vi "UHR-Fleezers Control (host) - Lorentz v5.vi"() -> ()   [LabVIEW 2014] (continued)
    n2967 = xnode "Get APD Data"("FPGA VI Reference In"=w4409, "error in"=w4408, "Number of Elements"=w4314, "Timeout (ms)"=-1) -> ("Data"=w4229:u32[], "Elements Remaining"=→"APD FIFO Elements Remaining":u32)  [unwired: 2 out]
    n2968 = feedback #1(0.0) -> (w4400:dbl)
    n2969 = To Time Stamp(1:w4400) -> (0:w4212:timestamp)
    n2970 = Add(x=w4235, y=w4400) -> (x+y=w4488:dbl)
    n2971 = feedback-in #1(w4488) -> ()
    n2972 = Subtract(x=w4513, y=w4444) -> (x-y=w4512:u32)
    n2973 = local read "APD Integration Time (s)"() -> (w4221:dbl)
    n2974 = Divide(x=w4511, y=w4512) -> (x/y=w4510:dbl)
    "Buffer Status" <- w4510
    n2975 = local read "Trap Sets"() -> (w4240:u32)
    n2976 = Equal?(x=w4510, y=1.0) -> (x = y?=w4508:bool)
    n2977 = local read "Number of APDs"() -> (w4228:u8)
    n2978 = Decimate 1D Array(w4377) -> (w4374:u16[], w4376:u16[], w4375:u16[], w4219:u16[], w4217:u16[])
    n2979 = case "Alert buffer overflow" shown="True" w4508 {
      frame False {
      }
      frame True {
        n2980 = call <vilib>:"Beep.vi"() -> ()  [unwired: 3 in, 9 out]
        "Overflow (data lost)" <- TRUE ("Overflow (data lost)")
      }
    }
    n2981 = To Unsigned Long Integer(number=w4374) -> (unsigned 32bit integer=w4373:u32[])
    n2982 = Join Numbers(hi=w4376, lo=w4375) -> ((hi.lo)=w4372:u32[])
    n2983 = Divide(x=w4219, y=w4218) -> (x/y=w4200:dbl[])
    n2984 = Divide(x=w4217, y=w4218) -> (x/y=w4199:dbl[])
    n2985 = call "deinterlace.vi"("Detector type"="Detector Type", "Data"=w4239, "Trap sets"=w4240, "Flip x sign"="Flip X Sign") -> ("Channel pattern"=w4236:i32, "Channel names"=w4172:string[], "Deinterlaced normalized data"=w4233:dbl[][], "Deinterlaced data"=w4237:i16[])
    "AI labels" <- w4172
    n2986 = Join Numbers(hi=w4373, lo=w4372) -> ((hi.lo)=w4367:u64[])
    n2987 = local read "Data Period (s)"() -> (w4206:dbl)
    n2988 = call "APD data extraction.vi"("Data"=w4229, "Number of APD's"=w4228, "APD integration time (s)"=w4221, "APD Ave N"="APD Ave N", "APD Disp. Downsample"="APD Disp. Downsample", "APD Disp. Scale"="APD Disp. Scale", "Time Stamp"=w4212) -> ("Output cluster"=→"APD rates cluster":T1, "Output Data"=w4224:T59, "Output waveform"=w4223:waveform(dbl)[], "APD Display period (s)"=w4222:dbl)
    "APD Display Period (s)" <- w4222
    n2989 = call "IR AOM word to freq - vec.vi"("Frequency Word In (double vec)"=w4367) -> ("Frequency Out"=w4404:dbl[])
    n2990 = Decimate 1D Array(w4199) -> (w4196:dbl[], w4195:dbl[])
    n2991 = Decimate 1D Array(w4200) -> (w4198:dbl[], w4197:dbl[])
    n2992 = Add(x=w4198, y=w4197) -> (x+y=w4194:dbl[])
    n2993 = Add(x=w4196, y=w4195) -> (x+y=w4193:dbl[])
    n2994 = Decimate 1D Array(w4404) -> (w4403:dbl[], w4402:dbl[])
    n2995 = Divide(x=w4194, y=w4192) -> (x/y=w4190:dbl[])
    n2996 = Divide(x=w4193, y=w4192) -> (x/y=w4191:dbl[])
    n2997 = Reciprocal(x=w4222) -> (1/x=→"APD Display Freq. (Hz)":dbl)
    n2998 = Build Array(w4403, w4402, w4190, w4191) -> (w4213:dbl[][])
    n2999 = Multiply(x=w4206, y="Trap Disp. Downsample") -> (x*y=w4401:dbl)
    "Display Period (s)" <- w4401
    n3000 = for {
      tunnel: w4233 -> [w4556] mode=indexing
      tunnel: [w4555] -> w4171 mode=indexing
      n3001 = call-poly <vilib>:"Mean.vi"("X"=w4556) -> ("mean"=w4555:dbl)  [unwired: 1 out]
    }
    "Values" <- w4171
    n3002 = call "Generate Waveform.vi"("Downsampling"="Trap Disp. Downsample", "Data Period (s)"=w4206, "Data"=w4233, "Plot names"=w4172, "Time Stamp"=w4212) -> ("Downsampled data"=w4231:waveform(dbl)[], "Non downsampled waveform"=w4230:waveform(dbl)[])
    n3003 = Multiply(x="APD Disp. Scale", y=w4223) -> (x*y=w4422:waveform(dbl)[])
    n3004 = Reciprocal(x=w4401) -> (1/x=→"Trap Disp. Freq. (Hz)":dbl)
    n3005 = Multiply(x="APD Disp. Downsample", y=w4221) -> (x*y=w4421:dbl)
    n3006 = Decimate 1D Array(w4237) -> (w4392:i16[], w4391:i16[], w4389:i16[], w4388:i16[])  [unwired: 9 out]
    n3007 = Divide(x=w4422, y=w4421) -> (x/y=w4319:waveform(dbl)[])
    n3008 = case shown="1" "Plot Trap Positions" {
      tunnel: [w4541 w4550] -> w4207
      frame 0, Default {
        n3009 = local read "BD 1 Frequency 2 (MHz)"() -> (w4544:dbl)
        n3010 = local read "BD 1 Frequency 1 (MHz)"() -> (w4545:dbl)
        n3011 = local read "T3 Y (V)"() -> (w4542:dbl)
        n3012 = local read "T3 X (V)"() -> (w4543:dbl)
        n3013 = Build Array(w4545, w4544, w4543, w4542) -> (w4541:dbl[])
      }
      frame 1 {
        w4549 = 75.0
        n3014 = Unbundle By Name("Piezo trap 0 position relative to 75 MHz") -> ("X (V)"=w4547:dbl, "Y (V)"=w4546:dbl)
        n3015 = Build Array(w4549, w4549, w4547, w4546) -> (w4550:dbl[])
      }
    }
    n3016 = Divide(x=w4392, y=w4391) -> (x/y=w4393:dbl[])
    n3017 = Divide(x=w4389, y=w4388) -> (x/y=w4390:dbl[])
    n3018 = local read "AOM X Cal (nm/MHz)"() -> (w4209:dbl)
    n3019 = Split 1D Array(array=w4393, index="N El. to Ave.") -> (second subarray=w4396:dbl[])  [unwired: 1 out]
    n3020 = Split 1D Array(array=w4390, index="N El. to Ave.") -> (second subarray=w4395:dbl[])  [unwired: 1 out]
    n3021 = Index Array(array=w4319, index=0) -> (element=w4417:waveform(dbl))
    n3022 = Index Array(array=w4319, index=1) -> (element=w4415:waveform(dbl))
    n3023 = Index Array(array=w4319, index=2) -> (element=w4321:waveform(dbl))
    n3024 = call-poly <vilib>:"Mean.vi"("X"=w4396) -> ("mean"=w4384:dbl)  [unwired: 1 out]
    n3025 = call-poly <vilib>:"Mean.vi"("X"=w4395) -> ("mean"=w4383:dbl)  [unwired: 1 out]
    n3026 = Subtract(x=w4417, y="APD 1 Offset") -> (x-y=w4413:waveform(dbl))
    n3027 = Subtract(x=w4415, y="APD 2 Offset") -> (x-y=w4412:waveform(dbl))
    n3028 = Subtract(x=w4321, y="APD 3 Offset") -> (x-y=w4318:waveform(dbl))
    n3029 = Build Array(w4413, w4412, w4318) -> (→"APD Chart":waveform(dbl)[])
    n3030 = Build Array(w4209, w4209, "Piezo Trap X cal (nm/V)", "Piezo Trap Y cal (nm/V)") -> (w4208:dbl[])
    n3031 = local read "Trap X AI1 (DMA)"() -> (w4394:T19)
    n3032 = To Fixed-Point(number=w4383) -> (fixed-point=w4381:fxp<+/-,16,1>)  [unwired: 1 in]
    n3033 = To Fixed-Point(number=w4384) -> (fixed-point=w4382:fxp<+/-,16,1>)  [unwired: 1 in]
    n3034 = Cluster To Array(cluster="Negate Axis") -> (array=w4201:bool[])
    n3035 = call "Generate Trap Positiion Waveform.vi"("Base trap positions"=w4207, "Data Period (s)"=w4206, "Input data"=w4213, "Position calibration values"=w4208, "Trap Pos. Disp. Downsample (s)"="Trap Pos. Disp. Downsample", "Negate axis"=w4201, "Time Stamp"=w4212) -> ("Output waveforms"=w4178:waveform(dbl)[])  [unwired: 3 in]
    "Trap Positions" <- w4178
    n3036 = Bundle By Name(cluster=w4394, "Set 1"=w4382, "Set 2"=w4381) -> (→"Trap X AI1 (DMA)":T19)
    n3037 = Initialize Array(0.0) -> (w4203:dbl[][])  [unwired: 2 in]
    n3038 = local read "Display Period (s)"() -> (w4431:dbl)
    n3039 = for {
      tunnel: w4178 -> [w4554] mode=indexing
      shift-right: [w4552] -> w4180
      shift-left: w4203 -> [w4553]
      n3040 = Unbundle By Name(w4554) -> ("Y"=w4551:dbl[])
      n3041 = Build Array (concatenate)(w4553, w4551) -> (w4552:dbl[][])
    }
    n3042 = Build Array (concatenate)(w4223, w4231) -> (w4234:waveform(dbl)[])
    "All Signals" <- w4234
    n3043 = Divide(x="Bead Sep. Int. Time (s)", y=w4431) -> (x/y=w4186:dbl)
    n3044 = feedback #2(w4180) -> (w4187:dbl[][])
    n3045 = call "Trap Pos RMS.vi"("Accumulated array"=w4187, "New Array"=w4180, "Number of sets to average"=w4186) -> ("Output accumulated array"=w4185:dbl[][], "RMS"=w4183:dbl[], "Mean"=w4184:dbl[])
    n3046 = feedback-in #2(w4185) -> ()
    n3047 = Index Array(array=w4180, index (row)=0 ("index")) -> (element=w4179:dbl[])  [unwired: 1 in]
    n3048 = Array To Cluster(array=w4183) -> (cluster=→"Trap RMS (ang)":T60)
    n3049 = Array To Cluster(array=w4184) -> (cluster=→"Mean Trap Positions (nm)":T61)
    n3050 = local read "Data points/scans (MCL)"() -> (w4471:dbl)
    n3051 = Unbundle(w4224) -> ("APD 1"=w4317:u32[])  [unwired: 2 out]
    n3052 = To Double Precision Float(number=w4317) -> (double precision float=w4439:dbl[])
    n3053 = Increment(x=w4471) -> (x+1=w4472:dbl)
    n3054 = feedback #3(w4472) -> (w4475:dbl)
    n3055 = Select(t=0, s=w4462, f=w4475) -> (s? t:f=w4468:dbl)
    n3056 = Array Size(array=w4439) -> (size(s)=w4474:i32)
    n3057 = Add(x=w4474, y=w4468) -> (x+y=w4469:dbl)
    n3058 = Greater?(x=w4469, y=w4471) -> (0:w4470:bool)
    n3059 = Select(t=w4468, s=w4470, f=w4469) -> (s? t:f=w4467:dbl)
    n3060 = feedback-in #3(w4467) -> ()
    n3061 = local read "MCL Scanning"() -> (w4465:bool)
    n3062 = Index Array(array=w4231, index="index 1") -> (element=w4309:waveform(dbl))
    n3063 = Index Array(array=w4231, index="index 2") -> (element=w4313:waveform(dbl))
    n3064 = Unbundle By Name(w4309) -> ("Y"=w4308:dbl[])
    n3065 = Unbundle By Name(w4313) -> ("Y"=w4312:dbl[])
    n3066 = Not(x=w4470) -> (.not. x?=w4464:bool)
    n3067 = And(x=w4464, y=w4465) -> (x .and. y?=w4466:bool)
    n3068 = call-poly <vilib>:"Mean.vi"("X"=w4308) -> ("mean"=→"Trap 1 sum mean":dbl)  [unwired: 1 out]
    n3069 = call-poly <vilib>:"Mean.vi"("X"=w4312) -> ("mean"=→"Trap 2 sum mean":dbl)  [unwired: 1 out]
    n3070 = Or(x=w4466, y=w4462) -> (x .or. y?=w4463:bool)
    n3071 = Equal?(x="Tab Control 6", y=T51."High Res Display") -> (x = y?=w4441:bool)
    n3072 = case shown="True" "X or Y?" {
      tunnel: w4231 -> [w4665 w4671]
      tunnel: [w4666 w4670] -> w4283
      tunnel: [w4664 w4669] -> w4280
      frame False {
        n3073 = Index Array(array=w4665, index=0) -> (element=w4666:waveform(dbl))
        n3074 = Index Array(array=w4665, index=3) -> (element=w4664:waveform(dbl))
      }
      frame True {
        n3075 = Index Array(array=w4671, index=1) -> (element=w4670:waveform(dbl))
        n3076 = Index Array(array=w4671, index=4) -> (element=w4669:waveform(dbl))
      }
    }
    n3077 = case "For displaying the high resolution display (no downsampling)" shown="True" w4441 {
      tunnel: w4230 -> [_ w4804]
      frame False {
      }
      frame True {
        n3078 = Index Array(array=w4804, index="High Res. Display") -> (element=w4805:waveform(dbl))
        n3079 = call <vilib>:"Std Deviation and Variance.vi"("X"=w4805) -> ("mean"=w4812:dbl, "standard deviation"=w4817:dbl)  [unwired: 1 in, 1 out]
        "Mean Intensity" <- w4812
        "Sigma" <- w4817
        n3080 = Subtract(x=w4805, y=w4812) -> (x-y=w4811:waveform(dbl))
        n3081 = Select(t=w4811, s="Subtract mean", f=w4805) -> (s? t:f=→"1 Channel":waveform(dbl))
        n3082 = Divide(x=w4817, y=w4812) -> (x/y=→"Sigma/Mean":dbl)
        n3083 = feedback #4(1) -> (w4806:i32)
        n3084 = Greater Or Equal?(x=w4806, y="Slow mean N ave.") -> (x >= y?=w4819:bool)
        n3085 = Increment(x=w4806) -> (x+1=w4821:i32)
        n3086 = Select(t=1, s=w4819, f=w4821) -> (s? t:f=w4808:i32)
        n3087 = feedback-in #4(w4808) -> ()
        n3088 = feedback #5() -> (w4809:waveform(dbl))  [unwired: 1 out]
        n3089 = case shown="Default" w4806 {
          tunnel: [w4824 w4827] -> w4810
          tunnel: w4809 -> [w4826 _]
          tunnel: w4805 -> [w4825 w4827]
          frame Default {
            n3090 = call-poly <vilib>:"Append Waveforms.vi"("waveform B"=w4825, "waveform A"=w4826) -> ("waveform out"=w4824:waveform(dbl))  [unwired: 1 in, 8 out]
          }
          frame 1 {
          }
        }
        n3091 = feedback-in #5(w4810) -> ()
        n3092 = case shown="True" w4819 {
          tunnel: w4810 -> [_ w4823]
          frame False {
          }
          frame True {
            n3093 = call-poly <vilib>:"Mean.vi"("X"=w4823) -> ("mean"=→"Slow mean":dbl)  [unwired: 1 out]
          }
        }
      }
    }
    n3094 = case "For plotting results of scanning MCL (fluorescence and detection laser images)" shown="True" w4463 {
      tunnel: w4462 -> [_ w4905]
      tunnel: w4471 -> [_ _]
      tunnel: w4230 -> [_ w5001]
      tunnel: w4410 -> [_ w4933]
      tunnel: w4224 -> [_ w4911]
      frame False {
      }
      frame True {
        w4874 = u32 0 items=["Horizontal", "Vertical", "Central", "1st Diagonal", "2nd Diagonal"] ("Type of Symmetry")
        w4878 = u32 0 items=["Horizontal", "Vertical", "Central", "1st Diagonal", "2nd Diagonal"] ("Type of Symmetry")
        w4879 = u32 0 items=["Horizontal", "Vertical", "Central", "1st Diagonal", "2nd Diagonal"] ("Type of Symmetry")
        w4880 = u32 0 items=["Horizontal", "Vertical", "Central", "1st Diagonal", "2nd Diagonal"] ("Type of Symmetry")
        w4884 = u32 0 items=["Horizontal", "Vertical", "Central", "1st Diagonal", "2nd Diagonal"] ("Type of Symmetry")
        # "Modified by Ronen \nbecause we do not have\nthe license for the\ntwo last image \nmanipulation VI's"
        n3095 = Unbundle(w4911) -> ("APD 1"=w4910:u32[], "APD 2"=w4908:u32[], "APD 3"=w4906:u32[])
        n3096 = To Double Precision Float(number=w4910) -> (double precision float=w4909:dbl[])
        n3097 = To Double Precision Float(number=w4908) -> (double precision float=w4907:dbl[])
        n3098 = To Double Precision Float(number=w4906) -> (double precision float=w4899:dbl[])
        n3099 = Index Array(array=w5001, index=10) -> (element=w5007:waveform(dbl))
        n3100 = Index Array(array=w5001, index=11) -> (element=w5004:waveform(dbl))
        n3101 = local read "Cycles/step (MCL)"() -> (w4963:u64)
        n3102 = Index Array(array=w5001, index="Channel") -> (element=w5003:waveform(dbl))
        n3103 = Unbundle(w4933) -> ("New Image"=w4932:T6, "New Image"=w4931:T6, "New Image"=w4912:T6, "New Image"=w4913:T6, "New Image"=w4914:T6)
        n3104 = local read "Scan steps (MCL)"() -> (w4901:u64)
        n3105 = Unbundle By Name(w5007) -> ("Y"=w4965:dbl[])
        n3106 = Unbundle By Name(w5004) -> ("Y"=w4967:dbl[])
        n3107 = local read "Scan lines (y)"() -> (w4902:u64)
        n3108 = local read "N APD Samp/step"() -> (w4904:dbl)
        n3109 = Unbundle By Name(w5003) -> ("Y"=w4972:dbl[])
        n3110 = call "downsample 1D array - double.vi"("Ave N"=w4963, "Array In"=w4965) -> ("Array Out"=w4964:dbl[])  [unwired: 1 out]
        n3111 = call "downsample 1D array - double.vi"("Ave N"=w4963, "Array In"=w4967) -> ("Array Out"=w4966:dbl[])  [unwired: 1 out]
        n3112 = call "downsample 1D array - double.vi"("Ave N"=w4963, "Array In"=w4972) -> ("Array Out"=w4971:dbl[])  [unwired: 1 out]
        n3113 = Multiply(x=w4901, y=u64 2) -> (x*y=w4903:u64)
        n3114 = feedback #6(w4907) -> (w4951:dbl[])
        n3115 = Build Array (concatenate)(w4951, w4907) -> (w4950:dbl[])
        n3116 = feedback #7(w4899) -> (w4900:dbl[])
        n3117 = Build Array (concatenate)(w4900, w4899) -> (w4898:dbl[])
        n3118 = Select(t=w4907, s=w4905, f=w4950) -> (s? t:f=w4935:dbl[])
        n3119 = feedback-in #6(w4935) -> ()
        n3120 = Select(t=w4899, s=w4905, f=w4898) -> (s? t:f=w4916:dbl[])
        n3121 = feedback-in #7(w4916) -> ()
        n3122 = feedback #8(w4909) -> (w5026:dbl[])
        n3123 = Build Array (concatenate)(w5026, w4909) -> (w5009:dbl[])
        n3124 = Select(t=w4909, s=w4905, f=w5009) -> (s? t:f=w5013:dbl[])
        n3125 = feedback-in #8(w5013) -> ()
        n3126 = feedback #9(w4964) -> (w5015:dbl[])
        n3127 = Build Array (concatenate)(w5015, w4964) -> (w5006:dbl[])
        n3128 = feedback #10(w4971) -> (w5024:dbl[])
        n3129 = Build Array (concatenate)(w5024, w4971) -> (w5023:dbl[])
        n3130 = feedback #11(w4966) -> (w5017:dbl[])
        n3131 = Build Array (concatenate)(w5017, w4966) -> (w5018:dbl[])
        n3132 = Select(t=w4964, s=w4905, f=w5006) -> (s? t:f=w4968:dbl[])
        n3133 = feedback-in #9(w4968) -> ()
        n3134 = Select(t=w4971, s=w4905, f=w5023) -> (s? t:f=w4970:dbl[])
        n3135 = feedback-in #10(w4970) -> ()
        n3136 = Select(t=w4966, s=w4905, f=w5018) -> (s? t:f=w4969:dbl[])
        n3137 = feedback-in #11(w4969) -> ()
        n3138 = call "integrate 1D array interval - double.vi"("Ave N"=w4904, "Array In"=w4935) -> ("Array Out"=w4946:dbl[])  [unwired: 1 out]
        n3139 = call "integrate 1D array interval - double.vi"("Ave N"=w4904, "Array In"=w4916) -> ("Array Out"=w4927:dbl[])  [unwired: 1 out]
        n3140 = call "integrate 1D array interval - double.vi"("Ave N"=w4904, "Array In"=w5013) -> ("Array Out"=w5012:dbl[])  [unwired: 1 out]
        n3141 = Array Size(array=w4946) -> (size(s)=w4947:i32)
        n3142 = Array Size(array=w4927) -> (size(s)=w4928:i32)
        n3143 = Array Size(array=w5012) -> (size(s)=w5014:i32)
        n3144 = Multiply(x=w4902, y=w4903) -> (x*y=w4949:u64)
        n3145 = Multiply(x=w4902, y=w4903) -> (x*y=w4930:u64)
        n3146 = Multiply(x=w4902, y=w4903) -> (x*y=w5022:u64)
        n3147 = Subtract(x=w4949, y=w4947) -> (x-y=w4940:u64)
        n3148 = call-poly <vilib>:"Mean.vi"("X"=w4946) -> ("mean"=w4937:dbl)  [unwired: 1 out]
        n3149 = Subtract(x=w4930, y=w4928) -> (x-y=w4921:u64)
        n3150 = call-poly <vilib>:"Mean.vi"("X"=w4927) -> ("mean"=w4918:dbl)  [unwired: 1 out]
        n3151 = Subtract(x=w5022, y=w5014) -> (x-y=w4962:u64)
        n3152 = call-poly <vilib>:"Mean.vi"("X"=w5012) -> ("mean"=w4959:dbl)  [unwired: 1 out]
        n3153 = call-poly <vilib>:"Mean.vi"("X"=w4968) -> ("mean"=w4952:dbl)  [unwired: 1 out]
        n3154 = call-poly <vilib>:"Mean.vi"("X"=w4970) -> ("mean"=w4957:dbl)  [unwired: 1 out]
        n3155 = call-poly <vilib>:"Mean.vi"("X"=w4969) -> ("mean"=w4955:dbl)  [unwired: 1 out]
        n3156 = Initialize Array(1.0 ("element"), w4940) -> (w4936:dbl[])
        n3157 = Initialize Array(1.0 ("element"), w4921) -> (w4917:dbl[])
        n3158 = Initialize Array(1.0 ("element"), w4962) -> (w4953:dbl[])
        n3159 = Multiply(x=w4936, y=w4937) -> (x*y=w4938:dbl[])
        n3160 = Multiply(x=w4917, y=w4918) -> (x*y=w4919:dbl[])
        n3161 = Multiply(x=w4953, y=w4959) -> (x*y=w4960:dbl[])
        n3162 = Multiply(x=w4953, y=w4955) -> (x*y=w4956:dbl[])
        n3163 = Multiply(x=w4953, y=w4957) -> (x*y=w4958:dbl[])
        n3164 = Multiply(x=w4953, y=w4952) -> (x*y=w4954:dbl[])
        n3165 = Build Array (concatenate)(w4946, w4938) -> (w4948:dbl[])
        n3166 = Build Array (concatenate)(w4927, w4919) -> (w4929:dbl[])
        n3167 = Build Array (concatenate)(w5012, w4960) -> (w5021:dbl[])
        n3168 = Build Array (concatenate)(w4968, w4954) -> (w5016:dbl[])
        n3169 = Build Array (concatenate)(w4970, w4958) -> (w5020:dbl[])
        n3170 = Build Array (concatenate)(w4969, w4956) -> (w5019:dbl[])
        n3171 = Reshape Array(w4948, w4902, w4903) -> (w4944:dbl[][])
        n3172 = Reshape Array(w4929, w4902, w4903) -> (w4925:dbl[][])
        n3173 = Reshape Array(w5021, w4902, w4903) -> (w4999:dbl[][])
        n3174 = Reshape Array(w5016, w4902, w4903) -> (w4982:dbl[][])
        n3175 = Reshape Array(w5020, w4902, w4903) -> (w4974:dbl[][])
        n3176 = Reshape Array(w5019, w4902, w4903) -> (w4989:dbl[][])
        n3177 = Array Subset(array=w4944, index (col)=0 ("index"), length (col)=w4901) -> (w4943:dbl[][])  [unwired: 2 in]
        n3178 = Array Subset(array=w4944, index (col)=w4901) -> (w4941:dbl[][])  [unwired: 3 in]
        n3179 = Array Subset(array=w4925, index (col)=0 ("index"), length (col)=w4901) -> (w4924:dbl[][])  [unwired: 2 in]
        n3180 = Array Subset(array=w4925, index (col)=w4901) -> (w4922:dbl[][])  [unwired: 3 in]
        n3181 = Array Subset(array=w4989, index (col)=0 ("index"), length (col)=w4901) -> (w4994:dbl[][])  [unwired: 2 in]
        n3182 = Array Subset(array=w4989, index (col)=w4901) -> (w4992:dbl[][])  [unwired: 3 in]
        n3183 = Array Subset(array=w4999, index (col)=0 ("index"), length (col)=w4901) -> (w4998:dbl[][])  [unwired: 2 in]
        n3184 = Array Subset(array=w4999, index (col)=w4901) -> (w4996:dbl[][])  [unwired: 3 in]
        n3185 = Array Subset(array=w4974, index (col)=0 ("index"), length (col)=w4901) -> (w4980:dbl[][])  [unwired: 2 in]
        n3186 = Array Subset(array=w4974, index (col)=w4901) -> (w4978:dbl[][])  [unwired: 3 in]
        n3187 = Array Subset(array=w4982, index (col)=0 ("index"), length (col)=w4901) -> (w4987:dbl[][])  [unwired: 2 in]
        n3188 = Array Subset(array=w4982, index (col)=w4901) -> (w4985:dbl[][])  [unwired: 3 in]
        n3189 = for {
          tunnel: w4943 -> [w5030] mode=indexing
          tunnel: [w5029] -> w4942 mode=indexing
          workers-P: _ -> [_]
          n3190 = Reverse 1D Array(array=w5030) -> (reversed array=w5029:dbl[])
        }
        n3191 = for {
          tunnel: w4924 -> [w5028] mode=indexing
          tunnel: [w5027] -> w4923 mode=indexing
          workers-P: _ -> [_]
          n3192 = Reverse 1D Array(array=w5028) -> (reversed array=w5027:dbl[])
        }
        n3193 = for {
          tunnel: w4994 -> [w5036] mode=indexing
          tunnel: [w5035] -> w4993 mode=indexing
          workers-P: _ -> [_]
          n3194 = Reverse 1D Array(array=w5036) -> (reversed array=w5035:dbl[])
        }
        n3195 = for {
          tunnel: w4998 -> [w5038] mode=indexing
          tunnel: [w5037] -> w4997 mode=indexing
          workers-P: _ -> [_]
          n3196 = Reverse 1D Array(array=w5038) -> (reversed array=w5037:dbl[])
        }
        n3197 = for {
          tunnel: w4980 -> [w5032] mode=indexing
          tunnel: [w5031] -> w4979 mode=indexing
          workers-P: _ -> [_]
          n3198 = Reverse 1D Array(array=w5032) -> (reversed array=w5031:dbl[])
        }
        n3199 = for {
          tunnel: w4987 -> [w5034] mode=indexing
          tunnel: [w5033] -> w4986 mode=indexing
          workers-P: _ -> [_]
          n3200 = Reverse 1D Array(array=w5034) -> (reversed array=w5033:dbl[])
        }
        n3201 = Index Array(array=w4999, index (row)=0) -> (element=→"Waveform Graph":dbl[])  [unwired: 1 in]
        n3202 = Add(x=w4942, y=w4941) -> (x+y=w4934:dbl[][])
        n3203 = Add(x=w4923, y=w4922) -> (x+y=w4915:dbl[][])
        n3204 = Add(x=w4993, y=w4992) -> (x+y=w4991:dbl[][])
        n3205 = Add(x=w4997, y=w4996) -> (x+y=w4973:dbl[][])
        n3206 = Add(x=w4979, y=w4978) -> (x+y=w4977:dbl[][])
        n3207 = Add(x=w4986, y=w4985) -> (x+y=w4984:dbl[][])
        n3208 = Divide(x=w4977, y=2) -> (x/y=w4975:dbl[][])
        n3209 = Divide(x=w4991, y=2) -> (x/y=w4892:dbl[][])
        n3210 = To Single Precision Float(number=w4973) -> (single precision float=w4896:sgl[][])
        n3211 = To Single Precision Float(number=w4934) -> (single precision float=w4891:sgl[][])
        n3212 = To Single Precision Float(number=w4915) -> (single precision float=w4890:sgl[][])
        n3213 = Divide(x=w4984, y=2) -> (x/y=w4893:dbl[][])
        n3214 = Transpose 2D Array(2D array=w4975) -> (transposed array=→"Data map":dbl[][])
        n3215 = To Single Precision Float(number=w4892) -> (single precision float=w4895:sgl[][])
        n3216 = To Single Precision Float(number=w4893) -> (single precision float=w4894:sgl[][])
        n3217 = call "IMAQ ArrayToImage"("Image Pixels (Float)"=w4896, "Image"=w4932) -> ("Image Out"=w4889:T6)  [unwired: 8 in, 1 out]
        n3218 = call "IMAQ ArrayToImage"("Image Pixels (Float)"=w4891, "Image"=w4931) -> ("Image Out"=w4888:T6)  [unwired: 8 in, 1 out]
        n3219 = call "IMAQ ArrayToImage"("Image Pixels (Float)"=w4890, "Image"=w4912) -> ("Image Out"=w4887:T6)  [unwired: 8 in, 1 out]
        n3220 = call "IMAQ ArrayToImage"("Image Pixels (Float)"=w4895, "Image"=w4913) -> ("Image Out"=w4886:T6)  [unwired: 8 in, 1 out]
        n3221 = call "IMAQ ArrayToImage"("Image Pixels (Float)"=w4894, "Image"=w4914) -> ("Image Out"=w4885:T6)  [unwired: 8 in, 1 out]
        n3222 = call "IMAQ Symmetry"("Type of Symmetry"=w4884, "Image Src"=w4889) -> ("Image Dst Out"=w4882:T6)  [unwired: 3 in, 1 out]
        n3223 = call "IMAQ Symmetry"("Type of Symmetry"=w4878, "Image Src"=w4888) -> ("Image Dst Out"=w4876:T6)  [unwired: 3 in, 1 out]
        n3224 = call "IMAQ Symmetry"("Type of Symmetry"=w4874, "Image Src"=w4887) -> ("Image Dst Out"=w4872:T6)  [unwired: 3 in, 1 out]
        n3225 = call "IMAQ Symmetry"("Type of Symmetry"=w4880, "Image Src"=w4886) -> ("Image Dst Out"=→"Detection Laser X":T6)  [unwired: 3 in, 1 out]
        n3226 = call "IMAQ Symmetry"("Type of Symmetry"=w4879, "Image Src"=w4885) -> ("Image Dst Out"=→"Detection Laser Y":T6)  [unwired: 3 in, 1 out]
        n3227 = call "IMAQ Set Simple Calibration"("Calibration Axis Info"=T52 {"Origin Pixel"={"X"=0.0, "Y"=0.0}, "Angle Relative to Horizontal (deg)"=0.0, "Axis Reference"=0}, "Grid Descriptor"=T53 {"X Step"=0.3, "Y Step"=0.3, "Unit"=enum."Undefined"}, "Image"=w4876) -> ("Calibrated Image"=→"APD 2":T6)  [unwired: 7 in, 1 out]
        n3228 = call "IMAQ Set Simple Calibration"("Calibration Axis Info"=T52 {"Origin Pixel"={"X"=0.0, "Y"=0.0}, "Angle Relative to Horizontal (deg)"=0.0, "Axis Reference"=0}, "Grid Descriptor"=T53 {"X Step"=0.3, "Y Step"=0.3, "Unit"=enum."Undefined"}, "Image"=w4872) -> ("Calibrated Image"=→"APD 3":T6)  [unwired: 7 in, 1 out]
        n3229 = call "IMAQ Set Simple Calibration"("Calibration Axis Info"=T52 {"Origin Pixel"={"X"=0.0, "Y"=0.0}, "Angle Relative to Horizontal (deg)"=0.0, "Axis Reference"=0}, "Grid Descriptor"=T53 {"X Step"=0.3, "Y Step"=0.3, "Unit"=enum."Undefined"}, "Image"=w4882) -> ("Calibrated Image"=→"APD 1":T6)  [unwired: 7 in, 1 out]
      }
    }
    n3230 = case "For computing FFTs for display" shown="True" "Compute FFT" {
      tunnel: w4230 -> [_ w5185]
      frame False {
      }
      frame True {
        n3231 = Build Array("FFT 1 Choice 1", "FFT 1 Choice 2", "FFT 2 Choice 1", "FFT 2 Choice 2") -> (w5178:u16[])
        n3232 = Array Size(array=w5185) -> (size(s)=w5184:i32)
        n3233 = feedback-in #12(w5178) -> ()
        n3234 = feedback #12(u16[] [100, 100, 100, 100]) -> (w5179:u16[])
        n3235 = feedback-in #13("# Spectra to Ave.") -> ()
        n3236 = feedback #13("# Spectra to Ave.") -> (w5176:dbl)
        n3237 = Not Equal?(x="# Spectra to Ave.", y=w5176) -> (x != y?=w5175:bool)
        n3238 = Not Equal?(x=w5178, y=w5179) -> (x != y?=w5177:bool)
        n3239 = feedback #14(1.0) -> (w5162:dbl)
        n3240 = Compound Arithmetic op=OR("Reset FFT", w5177, w5175) -> (w5160:bool)
        n3241 = Select(t=1.0, s=w5160, f=w5162) -> (s? t:f=w5164:dbl)
        n3242 = Greater?(x=w5164, y="# Spectra to Ave.") -> (0:w5183:bool)
        n3243 = Increment(x=w5164) -> (x+1=w5163:dbl)
        n3244 = feedback-in #14(w5163) -> ()
        n3245 = local read "DMA Update Period (s)"() -> (w5158:dbl)
        n3246 = Multiply(x="# Spectra to Ave.", y=w5158) -> (x*y=→"Ave. Time (s)":dbl)
        n3247 = Build Array(cluster{"f0":dbl, "df":dbl, "magnitude":dbl[]} {"f0"=0.0, "df"=0.0, "magnitude"=[]} ("PSD")) -> (w5167:cluster{"f0":dbl, "df":dbl, "magnitude":dbl[]}[])
        n3248 = Build Array(w5167, w5167, w5167, w5167) -> (w5169:T62)
        n3249 = feedback #15(w5169) -> (w5174:T62)
        n3250 = for {
          N: 4 -> [_]
          tunnel: w5178 -> [w5207] mode=indexing
          tunnel: w5185 -> [w5208]
          tunnel: w5184 -> [w5210]
          tunnel: w5160 -> [w5203]
          tunnel: w5183 -> [w5202]
          tunnel: "# Spectra to Ave." -> [w5201]
          tunnel: [w5200] -> w5173 mode=indexing
          tunnel: w5174 -> [w5205] mode=indexing
          tunnel: [w5204] -> w5161 mode=indexing
          tunnel: w5164 -> [w5199]
          n3251 = Less?(x=w5207, y=w5210) -> (x < y?=w5209:bool)
          n3252 = Index Array(array=w5208, index=w5207) -> (element=w5206:waveform(dbl))
          n3253 = case shown="True" w5209 {
            tunnel: w5206 -> [_ w5227]
            tunnel: w5205 -> [w5212 w5225]
            tunnel: [w5212 w5213] -> w5204
            tunnel: w5203 -> [_ w5224]
            tunnel: w5202 -> [_ w5217]
            tunnel: w5201 -> [_ w5216]
            tunnel: [cluster{"f0":dbl, "df":dbl, "magnitude":dbl[]} {"f0"=0.0, "df"=0.0, "magnitude"=[]} ("PSD") w5218] -> w5200
            tunnel: w5199 -> [_ w5215]
            frame False {
            }
            frame True {
              n3254 = call <vilib>:"Std Deviation and Variance.vi"("X"=w5227) -> ("mean"=w5228:dbl)  [unwired: 1 in, 2 out]
              n3255 = Subtract(x=w5227, y=w5228) -> (x-y=w5226:waveform(dbl))
              n3256 = xnode "Spectral Measurements"("Signals"=w5226) -> ("PSD"=w5220:cluster{"f0":dbl, "df":dbl, "magnitude":dbl[]})  [unwired: 1 in, 1 out]
              n3257 = case shown="False" w5224 {
                tunnel: w5225 -> [w5237 _]
                tunnel: [w5233 w5242] -> w5213
                tunnel: w5220 -> [w5236 w5243]
                tunnel: w5217 -> [w5235 _]
                frame False {
                  n3258 = Build Array (concatenate)(w5237, w5236) -> (w5234:cluster{"f0":dbl, "df":dbl, "magnitude":dbl[]}[])
                  n3259 = case shown="True" w5235 {
                    tunnel: w5234 -> [w5238 w5241]
                    tunnel: [w5238 w5239] -> w5233
                    frame False {
                    }
                    frame True {
                      n3260 = Delete From Array(array=w5241, index=0) -> (array with subset deleted=w5239:cluster{"f0":dbl, "df":dbl, "magnitude":dbl[]}[])  [unwired: 1 in, 1 out]
                    }
                  }
                }
                frame True {
                  n3261 = Build Array(w5243) -> (w5242:cluster{"f0":dbl, "df":dbl, "magnitude":dbl[]}[])
                }
              }
              n3262 = for {
                tunnel: w5213 -> [w5232] mode=indexing
                tunnel: [w5231] -> w5223 mode=indexing
                workers-P: _ -> [_]
                n3263 = Unbundle By Name(w5232) -> ("magnitude"=w5231:dbl[])
              }
              n3264 = Transpose 2D Array(2D array=w5223) -> (transposed array=w5222:dbl[][])
              n3265 = for {
                tunnel: w5222 -> [w5230] mode=indexing
                tunnel: [w5229] -> w5221 mode=indexing
                workers-P: _ -> [_]
                n3266 = Add Array Elements(numeric array=w5230) -> (sum=w5229:dbl)
              }
              n3267 = Select(t=w5216, s=w5217, f=w5215) -> (s? t:f=w5214:dbl)
              n3268 = Divide(x=w5221, y=w5214) -> (x/y=w5219:dbl[])
              n3269 = Bundle By Name(cluster=w5220, "magnitude"=w5219) -> (w5218:cluster{"f0":dbl, "df":dbl, "magnitude":dbl[]})
            }
          }
        }
        n3270 = case shown="True" w5160 {
          tunnel: w5161 -> [w5192 w5198]
          tunnel: [w5192 w5193] -> w5159
          frame False {
          }
          frame True {
            n3271 = Array Subset(array=w5198, index (row)=0 ("index"), length (row)=4 ("length"), index (col)=0 ("index"), length (col)=1 ("length")) -> (w5193:T62)
          }
        }
        n3272 = feedback-in #15(w5159) -> ()
        n3273 = Split 1D Array(array=w5173, index=2) -> (first subarray=→"FFT 1":cluster{"f0":dbl, "df":dbl, "magnitude":dbl[]}[], second subarray=→"FFT 2":cluster{"f0":dbl, "df":dbl, "magnitude":dbl[]}[])
      }
    }
    n3274 = local read "Offset Values"() -> (w4251:T20)
    n3275 = local read "T1 calibration"() -> (w4293:T9)
    n3276 = local read "T2 calibration"() -> (w4292:T8)
    n3277 = call-poly <vilib>:"Index Waveform Array.vi"("index"=16, "waveform array"=w4234) -> ("waveform"=w4268:waveform(dbl))  [unwired: 8 in, 1 out]
    n3278 = Unbundle By Name(w4283) -> ("Y"=w4291:dbl[])
    n3279 = Unbundle By Name(w4280) -> ("Y"=w4290:dbl[])
    n3280 = local read "Offset file step size"() -> (w4248:dbl)
    n3281 = Unbundle By Name(w4268) -> ("Y"=→"PSD Y Sum":dbl[])
    n3282 = call "calibrate trap data V2.vi"("Offset File step size"=w4248, "delta frequency"=w4250, "Dynamic offset update"="Dynamic offset\nupdate", "Offsets"=w4251, "T2 cal"=w4292, "T2"=w4290, "T1 cal"=w4293, "T1"=w4291) -> ("T2 force (pN)"=w4284:dbl[], "T2 position (nm)"=w4285:dbl[], "T1 force (pN)"=w4286:dbl[], "T1 position (nm)"=w4287:dbl[])
    n3283 = Bundle By Name(cluster=w4283, "Y"=w4287) -> (w4282:waveform(dbl))
    n3284 = Bundle By Name(cluster=w4283, "Y"=w4286) -> (w4281:waveform(dbl))
    n3285 = Bundle By Name(cluster=w4280, "Y"=w4285) -> (w4279:waveform(dbl))
    n3286 = Bundle By Name(cluster=w4280, "Y"=w4284) -> (w4278:waveform(dbl))
    n3287 = Subtract(x=w4287, y=w4285) -> (x-y=w4448:dbl[])
    n3288 = Negate(x=w4448) -> (-x=w4331:dbl[])
    n3289 = Subtract(x=w4331, y="Offset (nm)") -> (x-y=w4434:dbl[])
    n3290 = case "Choose calibrated display" shown="2" "Calibration" {
      tunnel: w4283 -> [w4861 _ _]
      tunnel: w4280 -> [w4860 _ _]
      tunnel: [w4861 w4863 w4865] -> w4263
      tunnel: [w4860 w4862 w4864] -> w4458
      tunnel: w4282 -> [_ w4863 _]
      tunnel: w4281 -> [_ _ w4865]
      tunnel: w4279 -> [_ w4862 _]
      tunnel: w4278 -> [_ _ w4864]
      frame 0, Default {
      }
      frame 1 {
      }
      frame 2 {
      }
    }
    n3291 = Bundle By Name(cluster=w4283, "Y"=w4434) -> (w4277:waveform(dbl))
    "Bead Separation" <- w4277
    n3292 = feedback #16(w4434) -> (w4433:dbl[])
    n3293 = Build Array (concatenate)(w4434, w4433) -> (w4288:dbl[])
    n3294 = Split 1D Array(array=w4288, index=w4186) -> (first subarray=w4289:dbl[])  [unwired: 1 out]
    n3295 = feedback-in #16(w4289) -> ()
    n3296 = Build Array(w4283, w4282, w4281, w4280, w4279, w4278, w4277) -> (w4276:waveform(dbl)[])
    n3297 = Not(x="Trap Trig. Fl.") -> (.not. x?=w4353:bool)
    n3298 = Unbundle By Name(w4263) -> ("Y"=w4332:dbl[])
    n3299 = Unbundle By Name(w4458) -> ("Y"=w4435:dbl[])
    n3300 = call-poly <vilib>:"Mean.vi"("X"=w4289) -> ("mean"=w4430:dbl)  [unwired: 1 out]
    "Bead Mean (nm)" <- w4430
    n3301 = Multiply(x=w4458, y=-1.0) -> (x*y=w4259:waveform(dbl))
    n3302 = call-poly <vilib>:"Mean.vi"("X"=w4332) -> ("mean"=w4335:dbl)  [unwired: 1 out]
    "T1 X" <- w4335
    n3303 = call-poly <vilib>:"Mean.vi"("X"=w4435) -> ("mean"=w4334:dbl)  [unwired: 1 out]
    "T2 X" <- w4334
    n3304 = Subtract(x=w4289, y=w4430) -> (x-y=w4429:dbl[])
    n3305 = Add(1:w4259, 2:w4263) -> (0:w4262:waveform(dbl))  [unwired: 1 in, 1 out]
    n3306 = Square(x=w4429) -> (x^2=w4428:dbl[])
    n3307 = Divide(x=w4262, y=2.0) -> (x/y=w4260:waveform(dbl))
    n3308 = Negate(x=w4435) -> (-x=w4301:dbl[])
    n3309 = call-poly <vilib>:"Mean.vi"("X"=w4428) -> ("mean"=w4427:dbl)  [unwired: 1 out]
    n3310 = Negate(x=w4334) -> (-x=w4333:dbl)
    n3311 = Square Root(x=w4427) -> (sqrt(x)=w4426:dbl)
    n3312 = Add(x=w4332, y=w4301) -> (x+y=w4436:dbl[])
    n3313 = Add(x=w4335, y=w4333) -> (x+y=w4454:dbl)
    n3314 = Multiply(x=10.0, y=w4426) -> (x*y=→"RMS (Ang)":dbl)
    n3315 = Divide(x=w4436, y=2.0) -> (x/y=w4304:dbl[])
    n3316 = Subtract(x=w4335, y=w4333) -> (x-y=→"Difference":dbl)
    n3317 = Build Array(w4263, w4259, w4260) -> (→"Force":waveform(dbl)[])
    n3318 = Select(t=w4301, s="Only check fixed trap T2", f=w4304) -> (s? t:f=→"Vec Mean of T1 T2":dbl[])
    n3319 = Divide(x=w4454, y=2.0) -> (x/y=w4245:dbl)
    "Mean" <- w4245
    n3320 = feedback-in #17("Trap Trig. Fl.") -> ()
    n3321 = feedback #17("Trap Trig. Fl.") -> (w4351:bool)
    n3322 = And(x=w4353, y=w4351) -> (x .and. y?=w4352:bool)
    n3323 = case "If have just turned off triggering" shown="True" w4352 {
      tunnel: w4256 -> [_ w4678]
      tunnel: w4347 -> [_ w4677]
      frame False {
      }
      frame True {
        w4676 = FALSE ("FPGA Trap Trig")
        n3324 = xnode "Read/Write Control"("FPGA VI Reference In"=w4678, "error in"=w4677, "FPGA Trap Trig"=w4676) -> ("FPGA VI Reference Out"=w4675:T35, "error out"=w4674:errorcluster)
        n3325 = xnode "Read/Write Control"("FPGA VI Reference In"=w4675, "error in"=w4674, "TTrig?"=w4676) -> ()  [unwired: 2 out]
        n3326 = local write "Initializing"(FALSE ("Initializing")) -> ()
        n3327 = local write "Triggered"(FALSE ("Triggered")) -> ()
        n3328 = local write "Waiting"(FALSE ("Waiting")) -> ()
      }
    }
    n3329 = Not(x=w4351) -> (.not. x?=w4364:bool)
    n3330 = And(x="Trap Trig. Fl.", y=w4364) -> (x .and. y?=w4361:bool)
    n3331 = Or(x=w4361, y="Reinitialize") -> (x .or. y?=w4350:bool)
    n3332 = feedback #18(w4357) -> (w4362:string)
    n3333 = Select(t=w4357, s=w4361, f=w4362) -> (s? t:f=w4356:string)
    n3334 = Select(t=w4357, s="Reinitialize", f=w4356) -> (s? t:f=w4355:string)
    n3335 = local read "Tether"() -> (w4438:bool)
    n3336 = feedback #19(0) -> (w4359:i32)
    n3337 = case "For determining if there is a tether still" shown="True" w4438 {
      tunnel: w4245 -> [_ w4787]
      frame False {
      }
      frame True {
        n3338 = Greater?(x="Lost Tether Alarm Threshold (pN)", y=w4787) -> (0:w4785:bool)
        n3339 = case shown="True" w4785 {
          frame False {
          }
          frame True {
            w4788 = FALSE ("Value (Signaling)")
            n3340 = flat-sequence {
              frame #0 {
                # "stop only if saving"
                n3341 = local read "Saving..."() -> (w4800:bool)
                n3342 = And(x=w4800, y="TA Cancel Save?") -> (x .and. y?=w4799:bool)
                n3343 = local write "Stop Saving"(w4799) -> ()
              }
              frame #1 {
                n3344 = case shown="True" "TA Green Off?" {
                  frame False {
                  }
                  frame True {
                    w4803 = FALSE ("Fl. Triggered...")
                    n3345 = local write "Fl. Triggered..."(w4803) -> ()
                    n3346 = property on="Green Laser ON" class="Bool (strict)"("Val(Sgnl)"=w4803) -> ()  [unwired: 2 in, 2 out]
                  }
                }
              }
            }
            n3347 = local read "Time tether formed"() -> (w4794:timestamp)
            n3348 = Get Date/Time In Seconds() -> (seconds since 1Jan1904=w4795:timestamp)
            n3349 = Subtract(x=w4795, y=w4794) -> (x-y=w4793:dbl)
            n3350 = Number To Decimal String(number=w4793) -> (decimal integer string=w4790:string)  [unwired: 1 out]
            n3351 = local read "Messages"() -> (w4797:string)
            n3352 = call <vilib>:"Beep.vi"() -> ()  [unwired: 3 in, 9 out]
            n3353 = Concatenate Strings("Lost tether (" ("Message to add"), w4790, " s)." ("string")) -> (w4792:string)
            n3354 = local write "Tether"(FALSE ("Tether")) -> ()
            n3355 = call "Update messages.vi"("Message to add"=w4792, "Old message string"=w4797) -> ("New message string"=w4796:string)
            n3356 = local write "Messages"(w4796) -> ()
            n3357 = property on="Fl. Triggered..." class="Bool (strict)"("Val(Sgnl)"=w4788) -> ()  [unwired: 2 in, 2 out]
            n3358 = local write "Dip for Protein"(w4788) -> ()
            n3359 = property on="Trap Pos. FB ON" class="Bool (strict)"("Val(Sgnl)"=w4788) -> ()  [unwired: 2 in, 2 out]
            n3360 = property on="Trap Trig. Fl." class="Bool (strict)"("Val(Sgnl)"=w4788) -> ()  [unwired: 2 in, 2 out]
          }
        }
      }
    }
    n3361 = case "For triggering actions based on the trap position (e.g., turning the excitation laser on if trap under feedback moves so far)" shown="True" "Trap Trig. Fl." {
      tunnel: w4179 -> [_ w4691]
      tunnel: w4355 -> [_ w4690]
      tunnel: ["" ("t") w4689] -> w4363
      tunnel: w4350 -> [_ w4688]
      tunnel: [0 ("t") w4687] -> w4360
      tunnel: w4359 -> [_ w4686]
      tunnel: w4256 -> [_ w4685]
      tunnel: w4347 -> [_ w4684]
      frame False {
      }
      frame True {
        n3362 = case shown="\"Wait for trigger\"" w4690 {
          tunnel: w4691 -> [w4708 _ _ w4756]
          tunnel: [w4705 w4737 "" ("t") w4759] -> w4689
          tunnel: w4688 -> [_ _ _ w4747]
          tunnel: [w4704 w4734 0 ("t") w4748] -> w4687
          tunnel: w4686 -> [_ w4736 _ w4754]
          tunnel: w4685 -> [w4693 w4731 _ w4750]
          tunnel: w4684 -> [w4692 w4730 _ w4749]
          frame "Wait for trigger" {
            n3363 = local read "Trap Trig. (FPGA)"() -> (w4696:bool)
            n3364 = Subtract(x=w4708, y="Mean T1 Position\nto compare (nm)") -> (x-y=w4701:dbl[])
            n3365 = call <vilib>:"Std Deviation and Variance.vi"("X"=w4701) -> ("mean"=→"mean":dbl, "standard deviation"=→"standard\ndeviation":dbl)  [unwired: 1 in, 1 out]
            n3366 = Array Max & Min(array=w4701) -> (max value=→"max value":dbl, min value=→"min value":dbl)  [unwired: 2 out]
            n3367 = Greater?(x=w4701, y="Threshold (nm)") -> (0:w4711:bool[])
            n3368 = case shown="True" w4696 {
              tunnel: w4693 -> [_ w4717]
              tunnel: w4692 -> [_ w4716]
              tunnel: [FALSE ("TTrig?") w4715] -> w4699
              frame False {
              }
              frame True {
                n3369 = xnode "Read/Write Control"("FPGA VI Reference In"=w4717, "error in"=w4716) -> ("TTrig?"=w4715:bool)  [unwired: 2 out]
              }
            }
            n3370 = Or Array Elements(Boolean array=w4711) -> (logical OR=w4698:bool)
            n3371 = Select(t=w4699, s=w4696, f=w4698) -> (s? t:f=w4697:bool)
            n3372 = Not(x=w4696) -> (.not. x?=w4695:bool)
            n3373 = And(x=w4697, y=w4695) -> (x .and. y?=w4694:bool)
            n3374 = Select(t="Triggered", s=w4697, f="Wait for trigger") -> (s? t:f=w4705:string)
            n3375 = case shown="True" w4697 {
              tunnel: [0 0] -> w4704
              tunnel: w4693 -> [_ w4722]
              tunnel: w4692 -> [_ w4721]
              frame False {
                "Waiting" <- TRUE ("Waiting")
              }
              frame True {
                n3376 = xnode "Read/Write Control"("FPGA VI Reference In"=w4722, "error in"=w4721, "TTrig?"=FALSE) -> ()  [unwired: 2 out]
                n3377 = local read "Messages"() -> (w4725:string)
                n3378 = call <vilib>:"Beep.vi"() -> ()  [unwired: 12 in]
                n3379 = call "Update messages.vi"("Message to add"="Unwinding trigger.", "Old message string"=w4725) -> ("New message string"=w4726:string)
                n3380 = local write "Messages"(w4726) -> ()
                n3381 = local write "Waiting"(FALSE ("Waiting")) -> ()
                "Triggered" <- TRUE ("Triggered")
              }
            }
            n3382 = case "Only need to turn on laser if host triggered" shown="True" w4694 {
              frame False {
              }
              frame True {
                n3383 = property on="Green Laser ON" class="Bool (strict)"("Val(Sgnl)"=TRUE ("Value (Signaling)")) -> ()  [unwired: 2 in, 2 out]
              }
            }
          }
          frame "Triggered" {
            n3384 = local read "Trap Trig. (FPGA)"() -> (w4733:bool)
            n3385 = Increment(x=w4736) -> (x+1=w4734:i32)
            n3386 = Greater Or Equal?(x=w4734, y="Fl. ON time (n)") -> (x >= y?=w4732:bool)
            n3387 = Select(t="Wait for trigger", s=w4732, f="Triggered" ("t")) -> (s? t:f=w4737:string)
            n3388 = And(x=w4732, y=w4733) -> (x .and. y?=w4729:bool)
            n3389 = case shown="True" w4729 {
              tunnel: w4731 -> [_ w4741]
              tunnel: w4730 -> [_ w4740]
              frame False {
              }
              frame True {
                n3390 = xnode "Read/Write Control"("FPGA VI Reference In"=w4741, "error in"=w4740, "FPGA Trap Trig"=TRUE) -> ()  [unwired: 2 out]
              }
            }
            n3391 = case shown="True" w4732 {
              frame False {
              }
              frame True {
                w4743 = FALSE ("Value (Signaling)")
                n3392 = local write "Triggered"(w4743) -> ()
                n3393 = local write "Waiting"(TRUE ("Waiting")) -> ()
                n3394 = property on="Green Laser ON" class="Bool (strict)"("Val(Sgnl)"=w4743) -> ()  [unwired: 2 in, 2 out]
              }
            }
          }
          frame "Do nothing" {
          }
          frame "Initialize", Default {
            n3395 = Increment(x=w4754) -> (x+1=w4758:i32)
            n3396 = Select(t=1, s=w4747, f=w4758) -> (s? t:f=w4748:i32)
            n3397 = feedback #20(w4756) -> (w4762:dbl[])
            n3398 = Build Array (concatenate)(w4756, w4762) -> (w4755:dbl[])
            n3399 = Greater Or Equal?(x=w4748, y="Wait to get offset (n)") -> (x >= y?=w4751:bool)
            n3400 = Select(t=w4756, s=w4747, f=w4755) -> (s? t:f=w4757:dbl[])
            n3401 = feedback-in #20(w4757) -> ()
            n3402 = call-poly <vilib>:"Mean.vi"("X"=w4757) -> ("mean"=w4752:dbl)  [unwired: 1 out]
            n3403 = local write "Mean T1 Position\nto compare (nm)"(w4752) -> ()
            n3404 = case shown="True" w4747 {
              tunnel: w4750 -> [_ w4768]
              tunnel: w4749 -> [_ w4767]
              frame False {
              }
              frame True {
                w4764 = FALSE ("FPGA Trap Trig")
                n3405 = xnode "Read/Write Control"("FPGA VI Reference In"=w4768, "error in"=w4767, "FPGA Trap Trig"=w4764) -> ("FPGA VI Reference Out"=w4766:T35, "error out"=w4765:errorcluster)
                n3406 = xnode "Read/Write Control"("FPGA VI Reference In"=w4766, "error in"=w4765, "TTrig?"=w4764) -> ()  [unwired: 2 out]
              }
            }
            n3407 = Select(t="Wait for trigger", s=w4751, f="Initialize") -> (s? t:f=w4759:string)
            n3408 = case shown="True" w4751 {
              tunnel: w4752 -> [_ w4771]
              tunnel: w4750 -> [_ w4780]
              tunnel: w4749 -> [_ w4779]
              frame False {
                n3409 = local write "Waiting"(FALSE ("Waiting")) -> ()
                "Initializing" <- TRUE ("Initializing")
              }
              frame True {
                n3410 = local read "Threshold (nm)"() -> (w4783:dbl)
                n3411 = local read "AOM X Cal (nm/MHz)"() -> (w4782:dbl)
                n3412 = Add(x=w4771, y=w4783) -> (x+y=w4784:dbl)
                n3413 = Divide(x=w4784, y=w4782) -> (x/y=w4781:dbl)
                n3414 = call "IR AOM freq to word.vi"("Frequency In (MHz)"=w4781) -> ("Frequency Word Out (double)"=w4778:dbl)
                n3415 = local write "Initializing"(FALSE ("Initializing")) -> ()
                n3416 = local write "Waiting"(TRUE ("Waiting")) -> ()
                n3417 = To Quad Integer(1:w4778) -> (0:w4777:i64)
                n3418 = xnode "Read/Write Control"("FPGA VI Reference In"=w4780, "error in"=w4779, "FPGA TTrig Thresh"=w4777) -> ("FPGA VI Reference Out"=w4774:T35, "error out"=w4773:errorcluster)
                n3419 = xnode "Read/Write Control"("FPGA VI Reference In"=w4774, "error in"=w4773, "FPGA Trap Trig"=TRUE) -> ()  [unwired: 2 out]
              }
            }
          }
        }
      }
    }
    n3420 = feedback-in #18(w4363) -> ()
    n3421 = feedback-in #19(w4360) -> ()
    n3422 = xnode ("Read/Write Control")("FPGA VI Reference In"=w4173, "error in"=w4446) -> ("FPGA VI Reference Out"=w4247:T35, "error out"=w4348:errorcluster, "AI2 Y Sum Set 1"=w4495:i16, "AI2 Y Sum Set 2"=w4494:i16, "AI1 X Set 1"=w4386:fxp<+/-,16,1>, "AI1 X Set 2"=w4385:fxp<+/-,16,1>, "Trap Pos FB Int Signal"=→"Trap Pos FB Int Signal":fxp<+/-,24,9>, "Trap Pos FB Int-Norm Signal"=→"Trap Pos FB Int-Norm Signal":fxp<+/-,16,1>, "Trap Pos FB Action"=w4379:i64, "Scanning"=→"AOD Scanning":bool, "Scan I"=→"AOD Scan I":u64, "Scanning MCL"=w4497:bool, "Scan I (MCL)"=→"MCL Scan I":u64, "Green FB Sum"=w4459:i16, "Trap Pos FB Action"=w4346:i64, "TTrig Fin Thresh"=w4342:i64, "Red FB Intensity"=w4329:i16, "Blue Intensity"=w4324:i16, "BD1 Frequency Out 1"=w4264:u64)
    "MCL Scanning" <- w4497
    "Trap Pos FB Action" <- w4379
    n3423 = Divide(x=w4329, y=3276.7) -> (x/y=w4328:dbl)
    "Red laser intensity (V)" <- w4328
    n3424 = Divide(x=w4324, y=3276.7) -> (x/y=w4323:dbl)
    "Blue laser intensity (V)" <- w4323
    n3425 = Divide(x=w4459, y=3276.7) -> (x/y=w4327:dbl)
    "Green laser intensity (V)" <- w4327
    n3426 = local read "FB Trig Integrate"() -> (w4340:u32)
    n3427 = Divide(x=w4346, y=w4340) -> (x/y=w4339:dbl)
    "TTrig Sig (Int)" <- w4339
    n3428 = Bundle(w4327, w4328, w4323) -> (→"Fluorescence laser intensities plot":cluster{dbl, dbl, dbl})  [unwired: 1 in]
    n3429 = Divide(x=w4342, y=w4340) -> (x/y=w4337:dbl)
    "TTrig Fin Thresh (Int)" <- w4337
    n3430 = local read "AOM X Cal (nm/MHz)"() -> (w4345:dbl)
    n3431 = local read "AI2 (V)"() -> (w4496:cluster{"Set 1":dbl, "Set 2":dbl})
    n3432 = Bundle By Name(cluster=w4496, "Set 1"=w4495, "Set 2"=w4494) -> (w4266:cluster{"Set 1":dbl, "Set 2":dbl})
    n3433 = Divide(x=w4379, y=327.67) -> (x/y=→"Action (%)":dbl)
    n3434 = case shown="True" "Semi Passive Mode" {
      tunnel: w4245 -> [_ w4561]
      frame False {
      }
      frame True {
        n3435 = local read "Target Force (pN)"() -> (w4559:dbl)
        n3436 = Less?(x="Jump Force (pN)", y=w4559) -> (x < y?=w4557:bool)
        n3437 = case shown="False" w4557 {
          tunnel: "Jump Force (pN)" -> [w4567 w4570]
          tunnel: w4561 -> [w4566 w4569]
          tunnel: [w4565 w4568] -> w4560
          frame False {
            n3438 = Less?(x=w4567, y=w4566) -> (x < y?=w4565:bool)
          }
          frame True {
            n3439 = Greater?(x=w4570, y=w4569) -> (0:w4568:bool)
          }
        }
        n3440 = case shown="False" w4560 {
          frame False {
            n3441 = local read "Trap Pos. FB ON"() -> (w4562:bool)
            n3442 = case shown="False" w4562 {
              frame False {
              }
              frame True {
                n3443 = property on="Trap Pos. FB ON" class="Bool (strict)"("Val(Sgnl)"=FALSE) -> ()  [unwired: 2 in, 2 out]
              }
            }
          }
          frame True {
            n3444 = property on="Trap Pos. FB ON" class="Bool (strict)"("Val(Sgnl)"=TRUE) -> ()  [unwired: 2 in, 2 out]
          }
        }
      }
    }
    n3445 = local read "Trap X (AI1)"() -> (w4399:T15)
    n3446 = call "IR AOM word double to freq.vi"("Frequency Word In (double)"=w4337) -> ("Frequency Out (MHz)"=w4336:dbl)
    n3447 = call "IR AOM word double to freq.vi"("Frequency Word In (double)"=w4339) -> ("Frequency Out (MHz)"=w4338:dbl)
    n3448 = Divide(x=w4266, y=3276.7) -> (x/y=w4492:cluster{"Set 1":dbl, "Set 2":dbl})
    n3449 = Multiply(x=w4338, y=w4345) -> (x*y=w4344:dbl)
    "TTrig Sig (nm)" <- w4344
    n3450 = Multiply(x=w4336, y=w4345) -> (x*y=w4343:dbl)
    "TTrig Fin Thresh (nm)" <- w4343
    n3451 = local write "AI2 (V)"(w4492) -> ()
    n3452 = Bundle(cluster=w4399, "Trap 1"=w4386, "Trap 2"=w4385) -> (→"Trap X (AI1)":T15)
    n3453 = local read "Trap Pos. FB ON"() -> (w4252:bool)
    n3454 = local read "Dynamic Force FB (ronen)"() -> (w4253:bool)
    n3455 = Bundle(w4344, w4343) -> (→"TTrig":cluster{dbl, dbl})  [unwired: 1 in]
    n3456 = Compound Arithmetic op=AND(w4253, "Real time Offset file correction for setpoint", w4252) -> (w4254:bool)
    n3457 = case shown="True" w4254 {
      tunnel: w4264 -> [_ _]
      tunnel: w4250 -> [_ w4589]
      tunnel: w4247 -> [_ w4572]
      frame False {
      }
      frame True {
        # "Changed by Ronen - real time update of set point\naccording to offset file"
        n3458 = local read "T1 calibration"() -> (w4584:T9)
        n3459 = local read "Offset file step size"() -> (w4591:dbl)
        n3460 = local read "Setpoint offset\ncorrection values"() -> (w4588:dbl[])
        n3461 = Multiply(x="Target Force (pN)", y=2.0) -> (x*y=w4585:dbl)
        n3462 = local read "Negate Diff?"() -> (w4573:bool)
        n3463 = Unbundle By Name(w4584) -> ("T1 alpha_x (nm/V)"=w4583:dbl, "T1 kappa_x (pN/nm)"=w4582:dbl)
        n3464 = Divide(x=w4589, y=w4591) -> (x/y=w4592:dbl)
        n3465 = To Long Integer(number=w4592) -> (32bit integer=w4590:i32)
        n3466 = Index Array(array=w4588, index=w4590) -> (element=w4575:dbl)
        n3467 = Multiply(x=w4583, y=w4582) -> (x*y=w4581:dbl)
        n3468 = Select(t=1, s=w4573, f=-1) -> (s? t:f=w4576:i32)
        n3469 = Divide(x=w4585, y=w4581) -> (x/y=w4580:dbl)
        n3470 = Multiply(x=w4576, y=w4575) -> (x*y=w4574:dbl)
        n3471 = Add(x=w4580, y=w4574) -> (x+y=w4579:dbl)
        n3472 = To Fixed-Point(number=w4579) -> (fixed-point=w4571:fxp<+/-,16,1>)  [unwired: 1 in]
        "Actual Setpoint" <- w4571
        n3473 = xnode "Read/Write Control"("FPGA VI Reference In"=w4572, "Trap Pos. FB SP"=w4571) -> ()  [unwired: 1 in, 2 out]
      }
    }
    n3474 = local read "All FB On/Off"() -> (w4265:bool)
    n3475 = case shown="True" w4265 {
      tunnel: w4266 -> [_ w4595]
      frame False {
      }
      frame True {
        n3476 = Divide(x=w4595, y=3276.7) -> (x/y=w4593:cluster{"Set 1":dbl, "Set 2":dbl})
        n3477 = Unbundle By Name(w4593) -> ("Set 1"=w4600:dbl, "Set 2"=w4599:dbl)
        n3478 = Greater?(x=w4600, y="Feedback Auto-Off threshold") -> (0:w4598:bool)
        n3479 = Greater?(x=w4599, y="Feedback Auto-Off threshold") -> (0:w4597:bool)
        n3480 = Or(x=w4598, y=w4597) -> (x .or. y?=w4596:bool)
        n3481 = case shown="True" w4596 {
          frame False {
          }
          frame True {
